vi "Out_S1F1.vi"(8 "error in (no error)":errorcluster, 11 "S1 Message Class in":refnum<class "S1 Message Class.lvclass">) -> (0 "error out":errorcluster, 3 "S1 Message Class out":refnum<class "S1 Message Class.lvclass">)   [LabVIEW 2020, in "SECS Communication.lvlib" / "S1 Message Class.lvclass"]
uses:
  S1 Message Class.lvclass
  D:/Dropbox/SECS/LabVIEW Code/Com/SECS Communication/SECS-II Class/SECS-II Class.lvclass
  S1 Message Class.lvclass/S1 Message Class.ctl
  SECS-II Class/SECS-II Class.lvclass
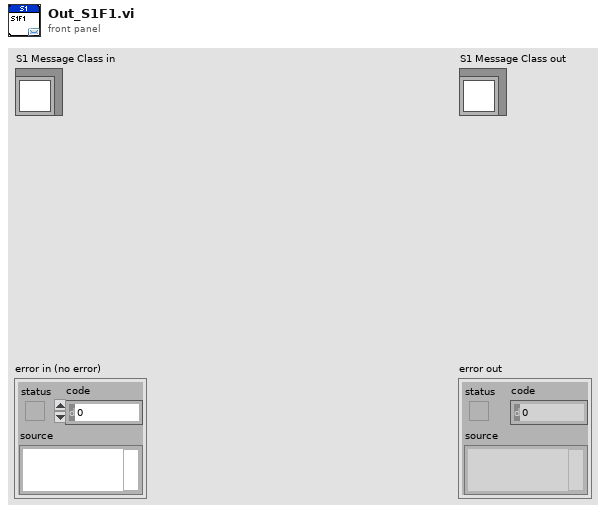
[diagram p1: front panel]
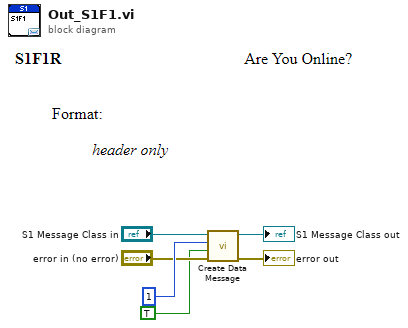
[diagram p0: block diagram]
diagram:
  n1 = call "Create Data Message.vi"("error in (no error)"="error in (no error)", "W-Bit"=TRUE, "Function"=u8 1, "SECS-II Class in"="S1 Message Class in") -> ("error out"=→"error out":errorcluster, "SECS-II Class out"=→"S1 Message Class out":refnum<class "S1 Message Class.lvclass">)  [unwired: 6 in]
